vi "GenerateNumericTankBoundariesWithHeater.vi"(3 "tank_resolution":T3, 5 "liquid":T1={"liquid_temperature"=array75x50[3750 elements], "water_level"=1.4948979591836733, "room_temperature"=298.15}, 6 "heater":T2={"heater_width"=0.5, "heater_heat"=50.0}) -> (0 "numeric_boundaries":cluster{dbl[][]}[](array[cluster]))   [LabVIEW 2020]
uses:
  TankResolution.ctl
  Heater.ctl
  Liquid.ctl
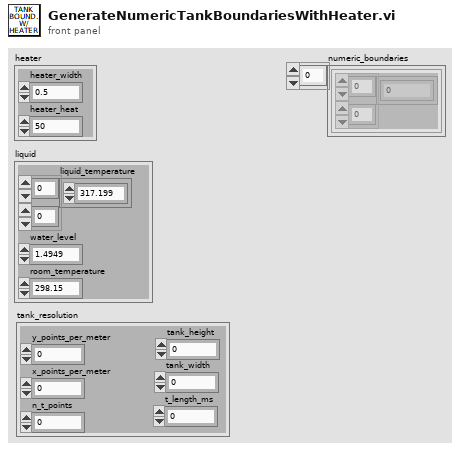
[diagram p1: front panel]
types:
  T1 = typedef "Liquid.ctl" = cluster{"liquid_temperature":dbl[][], "water_level":dbl, "room_temperature":dbl}
  T2 = typedef "Heater.ctl" = cluster{"heater_width":dbl, "heater_heat":dbl}
  T3 = typedef "TankResolution.ctl" = cluster{"y_points_per_meter":i32, "x_points_per_meter":i32, "n_t_points":i32, "tank_height":dbl, "tank_width":dbl, "t_length_ms":u32}
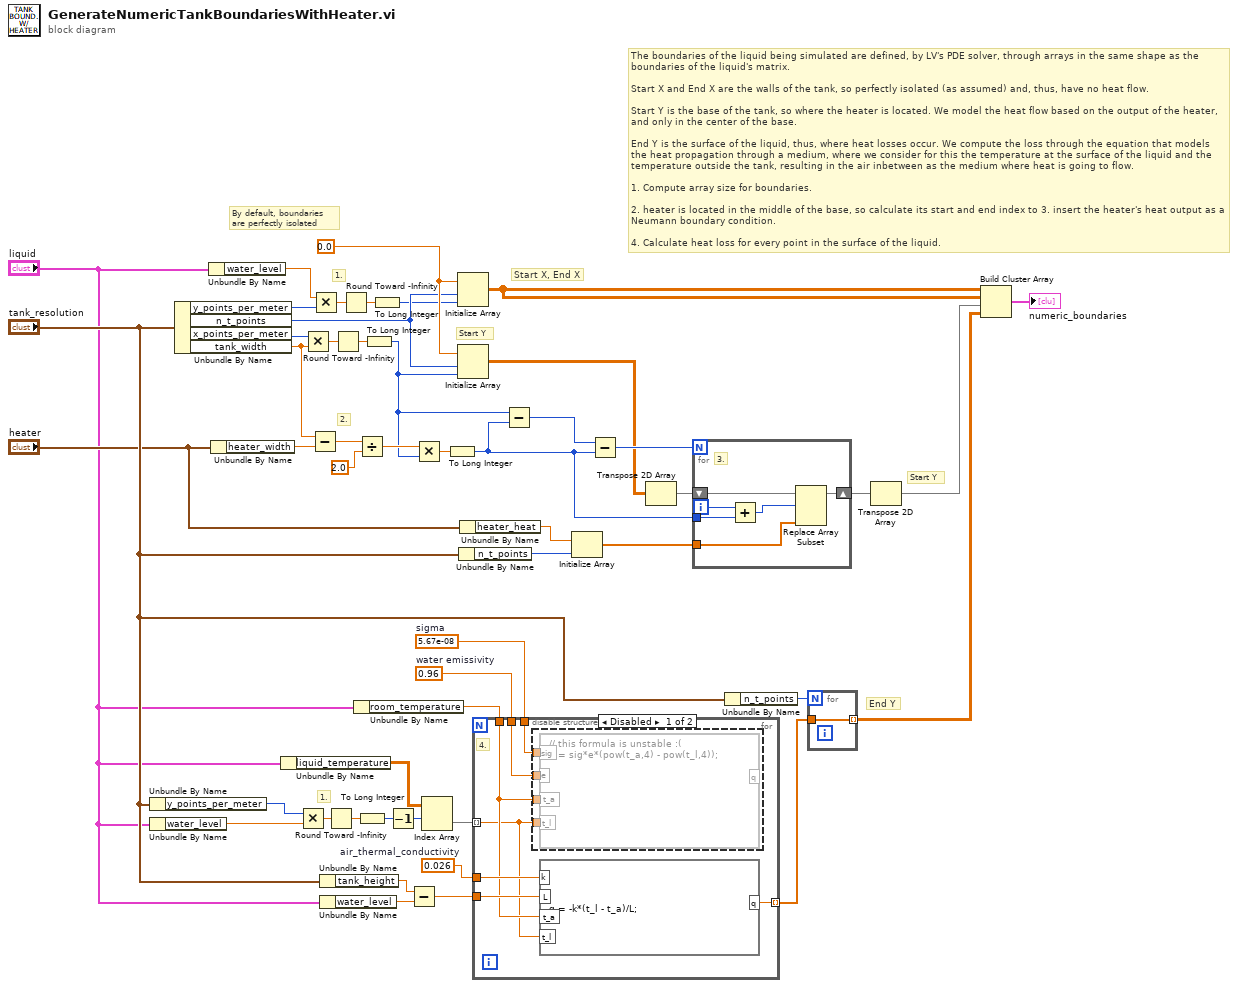
[diagram p0: block diagram]
diagram:
  w27 = 0.026  # air_thermal_conductivity
  w31 = 0.96  # water emissivity
  w32 = 5.67e-08  # sigma
  w43 = 0.0 ("element")
  # "1."
  # "2."
  # "1."
  # "The boundaries of the liquid being simulated are defined, by LV's PDE solver, through arrays in the same shape as the boundaries of the liquid's matrix.\n\nStart X and End X are the walls of the tank, so perfectly isolated (as assumed) and, thus, have no heat flow.\n\nStart Y is the base of the tank, so where the heater is located. We model the heat flow based on the output of the heater, and only in the center of the base.\n\nEnd Y is the surface of the liquid, thus, where heat losses occur. We compute the loss through the equation that models the heat propagation through a medium, where we consider for this the temperature at the surface of the liquid and the temperature outside the tank, resulting in the air inbetween as the medium where heat is going to flow.\n\n1. Compute array size for boundaries.\n\n2. heater is located in the middle of the base, so calculate its start and end index to 3. insert the heater's heat output as a Neumann boundary condition.\n\n4. Calculate heat loss for every point in the surface of the liquid."
  # "Start Y"
  # "End Y"
  # "Start Y"
  # "Start X, End X"
  # "By default, boundaries\nare perfectly isolated"
  n1 = Unbundle By Name("tank_resolution") -> ("y_points_per_meter"=w11:i32)
  n2 = Unbundle By Name("liquid") -> ("water_level"=w5:dbl)
  n3 = Unbundle By Name("tank_resolution") -> ("y_points_per_meter"=w24:i32, "n_t_points"=w35:i32, "x_points_per_meter"=w18:i32, "tank_width"=w16:dbl)
  n4 = Unbundle By Name("liquid") -> ("water_level"=w4:dbl)
  n5 = Unbundle By Name("heater") -> ("heater_width"=w10:dbl)
  n6 = Unbundle By Name("liquid") -> ("liquid_temperature"=w7:dbl[][])
  n7 = Multiply(x=w11, y=w5) -> (x*y=w14:dbl)
  n8 = Multiply(x=w18, y=w16) -> (x*y=w20:dbl)
  n9 = Subtract(x=w16, y=w10) -> (x-y=w49:dbl)
  n10 = Multiply(x=w4, y=w24) -> (x*y=w22:dbl)
  n11 = Unbundle By Name("tank_resolution") -> ("tank_height"=w15:dbl)
  n12 = Unbundle By Name("liquid") -> ("water_level"=w6:dbl)
  n13 = Round Toward -Infinity(1:w14) -> (0:w13:dbl)
  n14 = Round Toward -Infinity(1:w20) -> (0:w19:dbl)
  n15 = Round Toward -Infinity(1:w22) -> (0:w21:dbl)
  n16 = Unbundle By Name("liquid") -> ("room_temperature"=w3:dbl)
  n17 = Divide(x=w49, y=2.0) -> (x/y=w48:dbl)
  n18 = To Long Integer(number=w13) -> (32bit integer=w12:i32)
  n19 = To Long Integer(number=w19) -> (32bit integer=w17:i32)
  n20 = To Long Integer(number=w21) -> (32bit integer=w23:i32)
  n21 = Decrement(x=w12) -> (x-1=w34:i32)
  n22 = Subtract(x=w15, y=w6) -> (x-y=w25:dbl)
  n23 = Multiply(x=w48, y=w17) -> (x*y=w47:dbl)
  n24 = Index Array(array=w7, index (row)=w34) -> (element=w33:dbl[])  [unwired: 1 in]
  n25 = To Long Integer(number=w47) -> (32bit integer=w1:i32)
  n26 = Initialize Array(w43, w35, w23) -> (w42:dbl[][])
  n27 = Initialize Array(w43, w35, w17) -> (w37:dbl[][])
  n28 = Unbundle By Name("tank_resolution") -> ("n_t_points"=w36:i32)
  n29 = Unbundle By Name("heater") -> ("heater_heat"=w9:dbl)
  n30 = for {
    tunnel: w33 -> [w51] mode=indexing
    tunnel: w32 -> [w57]
    tunnel: w31 -> [w56]
    tunnel: w3 -> [w52]
    tunnel: [w55] -> w29 mode=indexing
    tunnel: w27 -> [w54]
    tunnel: w25 -> [w53]
    # "4."
    n31 = disable-structure shown="Disabled" {
      disable-tunnel: w57 -> [w61 _]
      disable-tunnel: w56 -> [w60 _]
      disable-tunnel: w52 -> [w59 _]
      disable-tunnel: w51 -> [w58 _]
      frame Disabled {
        n32 = formula code="// this formula is unstable :(\nq = sig*e*(pow(t_a,4) - pow(t_l,4));"("sig"=w61, "e"=w60, "t_a"=w59, "t_l"=w58) -> ()  [unwired: 1 out]
      }
      frame Enabled {
      }
    }
    n33 = formula code="q = -k*(t_l - t_a)/L;"("k"=w54, "L"=w53, "t_a"=w52, "t_l"=w51) -> ("q"=w55:dbl)
  }
  n34 = Subtract(x=w17, y=w1) -> (x-y=w46:i32)
  n35 = Initialize Array(w9, w36) -> (w44:dbl[])
  n36 = Subtract(x=w46, y=w1) -> (x-y=w45:i32)
  n37 = Transpose 2D Array(2D array=w37) -> (transposed array=w40:dbl[][])
  n38 = for {
    N: w45 -> [_]
    shift-right: [w66] -> w39
    shift-left: w40 -> [w67]
    tunnel: w1 -> [w64]
    tunnel: w44 -> [w62]
    i -> [w65]
    # "3."
    n39 = Add(x=w65, y=w64) -> (x+y=w63:i32)
    n40 = Replace Array Subset(array=w67, new element=w62, index (row)=w63) -> (w66:dbl[][])  [unwired: 1 in]
  }
  n41 = Unbundle By Name("tank_resolution") -> ("n_t_points"=w30:i32)
  n42 = for {
    N: w30 -> [_]
    tunnel: [w68] -> w28 mode=indexing
    tunnel: w29 -> [w68]
  }
  n43 = Transpose 2D Array(2D array=w39) -> (transposed array=w38:dbl[][])
  n44 = Build Cluster Array(w42, w42, w38, w28) -> (→"numeric_boundaries":cluster{dbl[][]}[])
